vi "Smoke Alarm.vi"() -> ()   [LabVIEW 2024]
uses:
  <vilib>/Instr/_visa.llb/VISA Configure Serial Port (Instr).vi
panel:
  out "Boolean":bool
  in  "STOP":bool
  out "?":i32(graph)
  out "GAS LEVEL":i32
  in  "?":refnum<visa-resource-name>
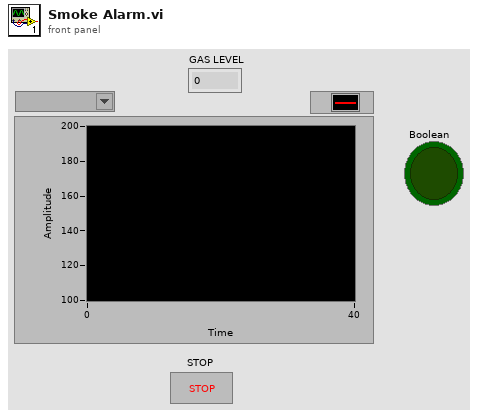
[diagram p1: front panel]
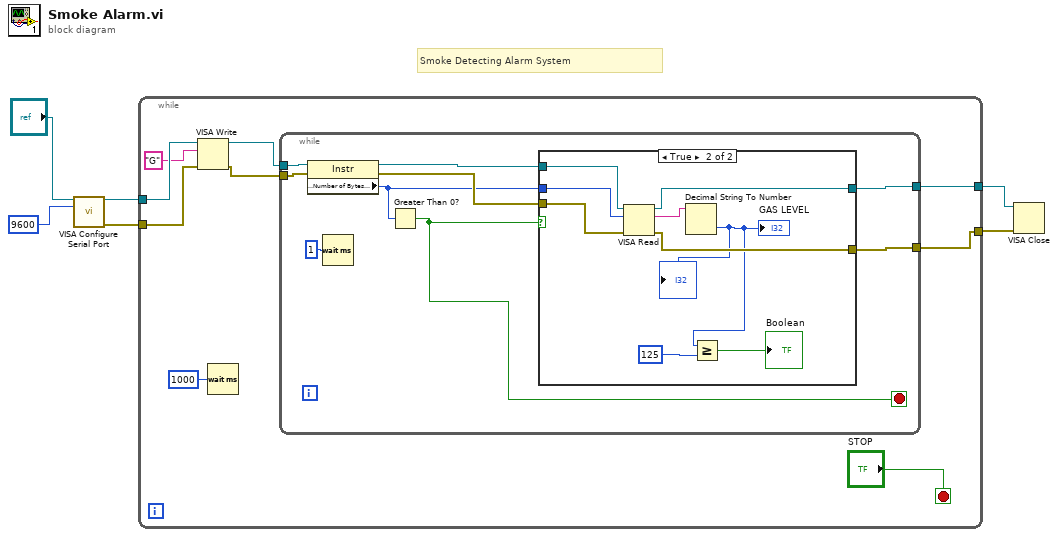
[diagram p0: block diagram]
diagram:
  # "Smoke Detecting Alarm System"
  n1 = call-poly "VISA Configure Serial Port"("VISA resource name"="?", "baud rate (9600)"=u32 9600) -> ("VISA resource name out"=w4:refnum<visa-resource-name>, "error out"=w3:errorcluster)  [unwired: 12 in]
  n2 = while {
    tunnel: w4 -> [w15]
    tunnel: w3 -> [w14]
    tunnel: [w9] -> w1
    tunnel: [w8] -> w2
    stop <- "STOP" stop-if-true
    n3 = VISA Write(VISA resource name=w15, write buffer="G", error in (no error)=w14) -> (VISA resource name out=w12:refnum<visa-resource-name>, error out=w11:errorcluster)  [unwired: 1 out]
    n4 = Wait (ms)(milliseconds to wait=u32 1000) -> ()  [unwired: 1 out]
    n5 = while {
      tunnel: w12 -> [w24]
      tunnel: w11 -> [w23]
      tunnel: [w19] -> w9
      tunnel: [w18] -> w8
      stop <- w16 stop-if-true
      n6 = property class="Instr"(reference=w24, error in=w23) -> (reference out=w22:refnum<visa-resource-name>, error out=w21:errorcluster, "Serial Settings:Number of Bytes at Serial Port"=w20:u32)
      n7 = Wait (ms)(milliseconds to wait=u32 1) -> ()  [unwired: 1 out]
      n8 = Greater Than 0?(x=w20) -> (x > 0?=w16:bool)
      n9 = case shown="True" w16 {
        tunnel: w22 -> [w26 w35]
        tunnel: w21 -> [w25 w34]
        tunnel: w20 -> [_ w33]
        tunnel: [w26 w31] -> w19
        tunnel: [w25 w30] -> w18
        frame False {
        }
        frame True {
          n10 = VISA Read(VISA resource name=w35, byte count=w33, error in (no error)=w34) -> (VISA resource name out=w31:refnum<visa-resource-name>, read buffer=w32:string, error out=w30:errorcluster)  [unwired: 1 out]
          n11 = Decimal String To Number(string=w32) -> (number=w28:i32)  [unwired: 2 in, 1 out]
          "GAS LEVEL" <- w28
          "?" <- w28
          n12 = Greater Or Equal?(x=w28, y=125) -> (x >= y?=→"Boolean":bool)
        }
      }
    }
  }
  n13 = VISA Close(VISA resource name=w1, error in (no error)=w2) -> ()  [unwired: 1 out]
